vi "VFD.vi"() -> (0 "GS1 Communication Error Out":errorcluster)   [LabVIEW 2017]
uses:
  XDataNode.xnode
panel:
  in  "GS1 Communication Error In":errorcluster
  out "Iteration Duration":i64
  out "Finished Late? [i-1]":bool
  out "TCHX Initializaton Error":errorcluster
  out "TCHX Initialization Loop Time (ms)":u32
  out "CTAH Initializaton Error":errorcluster
  out "CTAH Initialization Loop Time (ms)":u32
  out "Pump Initializaton Error":errorcluster
  out "Pump Initialization Loop Time (ms)":u32
  in  "Starting Address":u16
  out "Holding Registers":u16[](array[numeric])
  out "error out":errorcluster
  out "VISA resource name out":refnum<visa-resource-name>
  out "400001":u16
  out "error out":errorcluster
  # "Troubleshooting Modbus communication using third-party VIs and native I/O Server"
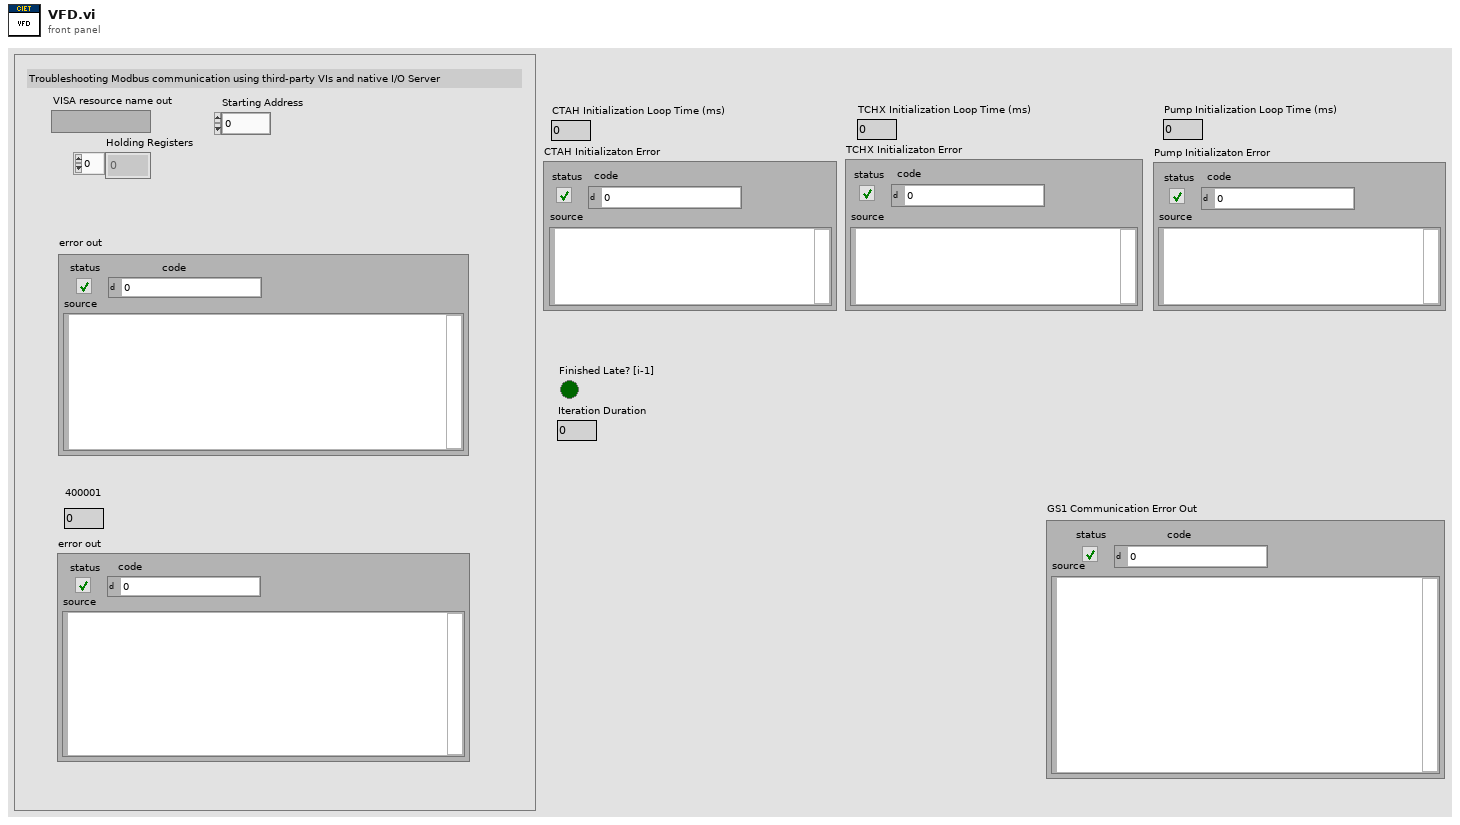
[diagram p1: front panel]
types:
  T1 = cluster{"Mode":enum16{"RTU", "ASCII"}, "Slave Address":u8}
  T2 = cluster{"Expected End [f-1]":u64, "Actual End [f-1]":u64, "Finished Late? [f-1]":bool, "Expected End [i-1]":u64, "Actual End [i-1]":u64, "Finished Late? [i-1]":bool, "Expected Start [i]":u64, "Actual Start [i]":u64, "Expected Start [f]":u64, "Actual Start [f]":u64, "Source Name":string, "Structure Name":string, "Period":i64, "Deadline":i64, "Offset":i64, "Start":i64, "Priority":i32, "Timeout":i32, "Mode":enum32{"No Change", "Process missed periods, maintain original phase", "Discard missed periods, maintain original phase", "Process missed periods, ignore original phase", "Discard missed periods, ignore original phase"}, "Wakeup Reason":enum32{"Normal", "Aborted", "Asynchronous wakeup", "Timing source error", "Timed loop error", "Timeout"}, "Error":errorcluster, "Source Type":string, "Secondary Source Type":string, "Global End Time":u64, "Global Start Time":u64, "Frame Duration":u64, "Iteration Duration":u64, "Assigned CPU":i32, "I/O Scan Engine Mode":u32}
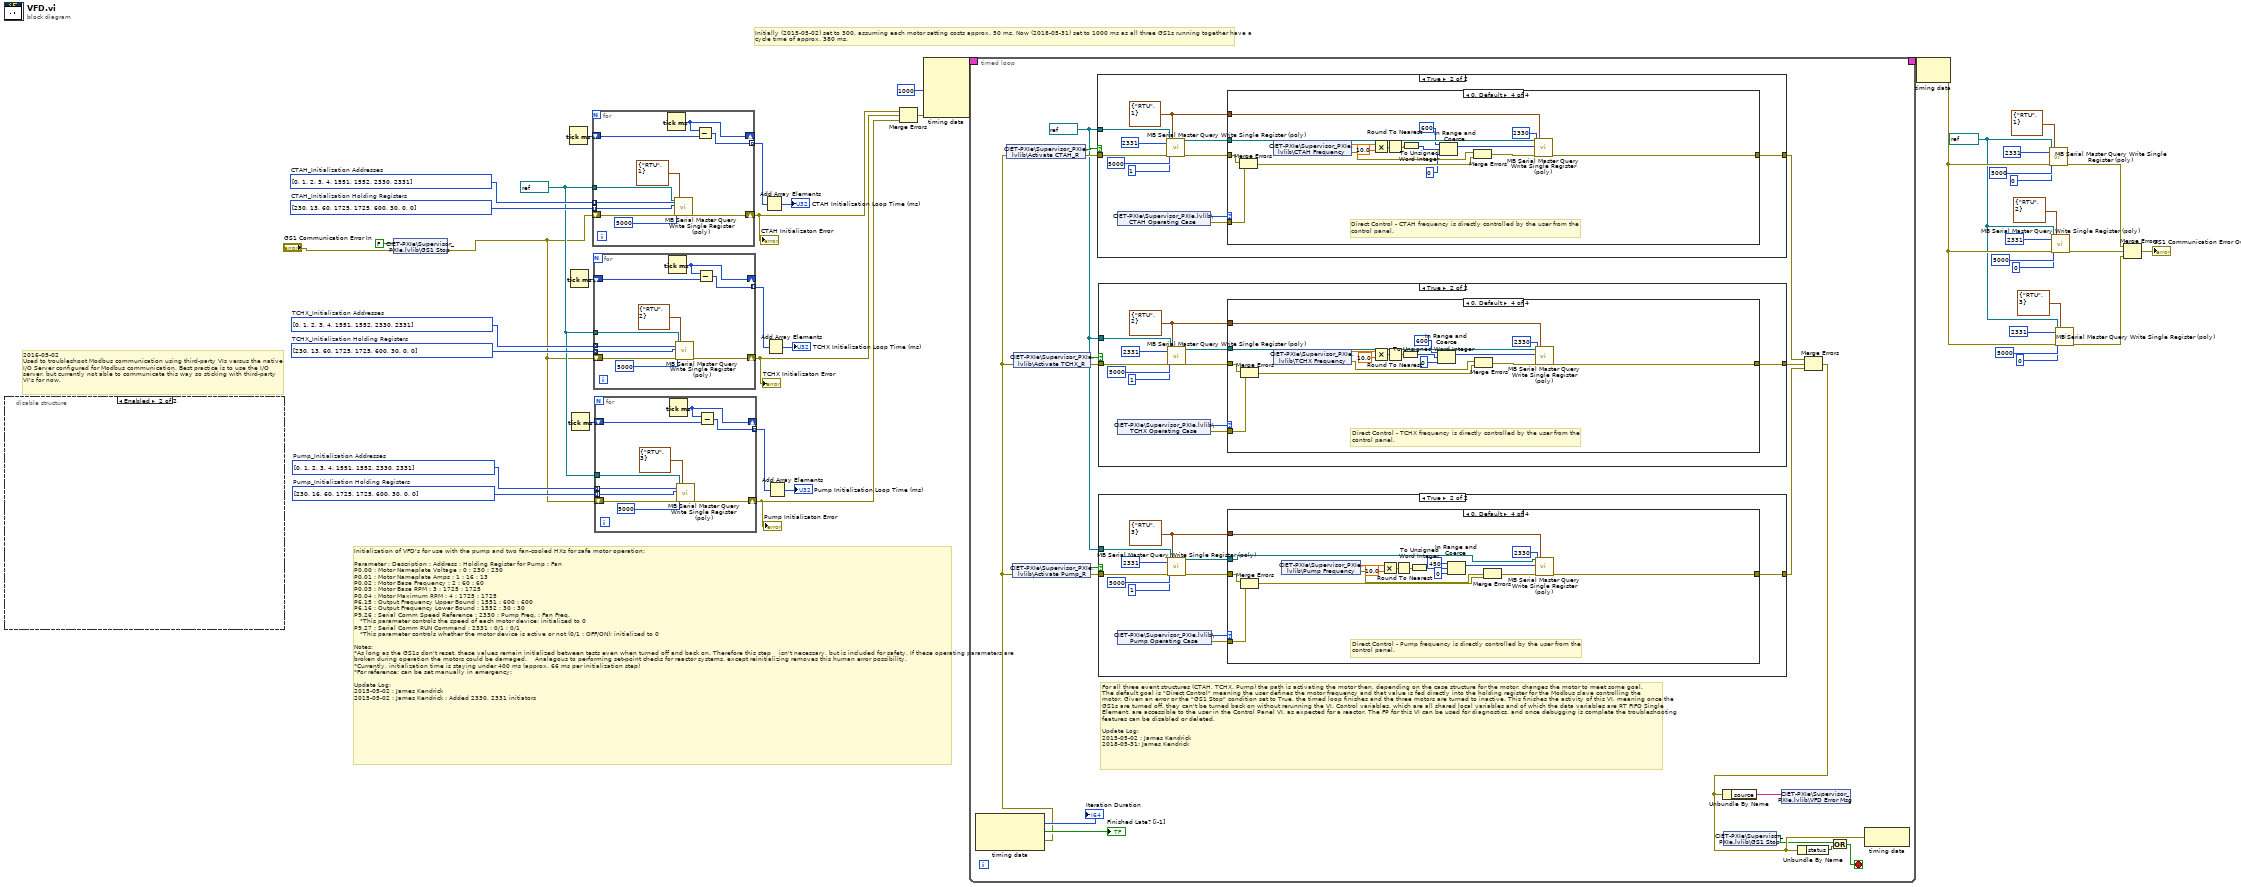
[diagram p0: block diagram]
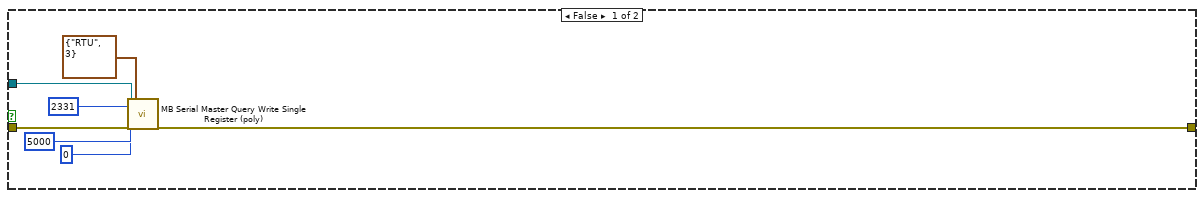
[diagram p2: hidden frame]
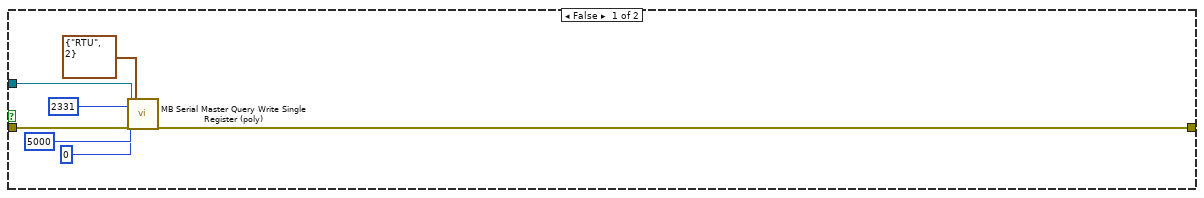
[diagram p6: hidden frame]
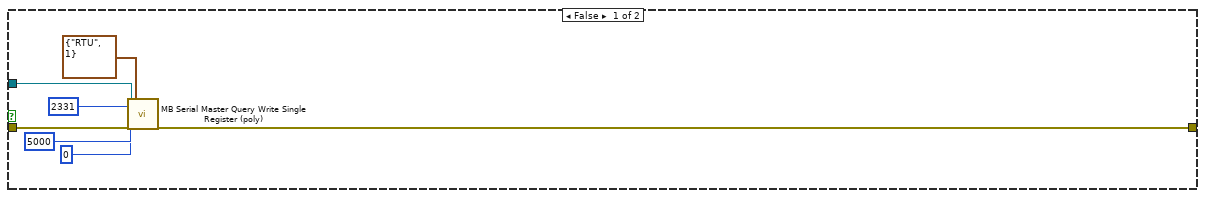
[diagram p10: hidden frame]
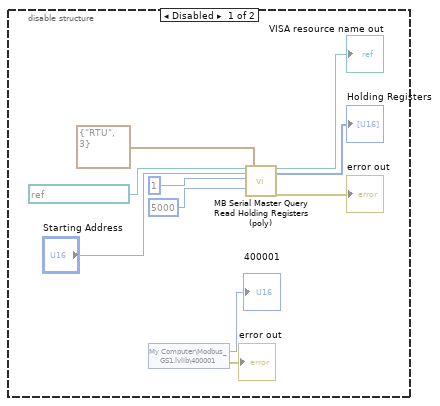
[diagram p14: hidden frame]
diagram:
  w7 = refnum<visa-resource-name> "VFD" ("VISA resource name")
  w8 = refnum<visa-resource-name> "VFD" ("VISA resource name")
  w30 = u16[] [230, 13, 60, 1725, 1725, 600, 30, 0, 0]  # TCHX_Initialization Holding Registers
  w31 = u16[] [0, 1, 2, 3, 4, 1551, 1552, 2330, 2331]  # TCHX_Initialization Addresses
  w35 = u16[] [230, 13, 60, 1725, 1725, 600, 30, 0, 0]  # CTAH_Initialization Holding Registers
  w36 = u16[] [0, 1, 2, 3, 4, 1551, 1552, 2330, 2331]  # CTAH_Initialization Addresses
  w43 = u16[] [230, 16, 60, 1725, 1725, 600, 30, 0, 0]  # Pump_Initialization Holding Registers
  w44 = u16[] [0, 1, 2, 3, 4, 1551, 1552, 2330, 2331]  # Pump_Initialization Addresses
  # "Initially (2015-05-02) set to 300, assuming each motor setting costs approx. 50 ms. Now (2018-05-31) set to 1000 ms as all three GS1s running together have a \ncycle time of approx. 380 ms."
  # "2016-05-02\nUsed to troubleshoot Modbus communication using third-party VIs versus the native\nI/O Server configured for Modbus communication. Best practice is to use the I/O \nserver, but currently not able to communicate this way so sticking with third-party \nVI's for now."
  # "Initialization of VFD's for use with the pump and two fan-cooled HXs for safe motor operation:\n\nParameter : Description : Address : Holding Register for Pump : Fan\nP0.00 : Motor Nameplate Voltage : 0 : 230 : 230\nP0.01 : Motor Nameplate Amps : 1 : 16 : 13\nP0.02 : Motor Base Frequency : 2 : 60 : 60\nP0.03 : Motor Base RPM : 3 : 1725 : 1725\nP0.04 : Motor Maximum RPM : 4 : 1725 : 1725\nP6.15 : Output Frequency Upper Bound : 1551 : 600 : 600\nP6.16 : Output Frequency Lower Bound : 1552 : 30 : 30\nP9.26 : Serial Comm Speed Reference : 2330 : Pump Freq. : Fan Freq. \n   *This parameter controls the speed of each motor device; initialized to 0\nP9.27 : Serial Comm RUN Command : 2331 : 0/1 : 0/1\n   *This parameter controls whether the motor device is active or not (0/1 : OFF/ON); initialized to 0\n\nNotes:\n*As long as the GS1s don't reset, these values remain initialized between tests even when turned off and back on. Therefore this step    isn't necessary, but is included for safety. If these operating parameters are broken during operation the motors could be damaged.    Analagous to performing set-point checks for reactor systems, except reinitializing removes this human error possibility.\n*Currently, initialization time is staying under 400 ms (approx. 66 ms per initialization step)\n*For reference; can be set manually in emergency:\n\nUpdate Log:\n2015-05-02 : James Kendrick \n2015-05-02 : James Kendrick : Added 2330, 2331 initiators"
  n1 = disable-structure shown="Enabled" {
    frame Disabled {
      n2 = shared-variable "My Computer\\Modbus_GS1.lvlib\\400001"() -> (→"400001":u16, error out=→"error out":errorcluster)  [unwired: 1 in]
      n3 = call "MB Serial Master Query Read Holding Registers (poly).vi"("VISA resource name"=refnum<visa-resource-name> "GS1_AC_Drive", "Starting Address"="Starting Address", "Quantity"=u16 1, "Timeout"=u32 5000, "Serial Parameters"=T1 {"Mode"=enum."RTU", "Slave Address"=3}) -> ("VISA resource name out"=→"VISA resource name out":refnum<visa-resource-name>, "Holding Registers"=→"Holding Registers":u16[], "error out"=→"error out":errorcluster)  [unwired: 11 in, 1 out]
    }
    frame Enabled {
    }
  }
  n4 = shared-variable "CIET-PXIe\\Supervisor_PXIe.lvlib\\GS1 Stop"(FALSE ("GS1 Stop"), error in="GS1 Communication Error In") -> (error out=w2:errorcluster)
  n5 = Tick Count (ms)() -> (millisecond timer value=w34:u32)
  n6 = Tick Count (ms)() -> (millisecond timer value=w29:u32)
  n7 = Tick Count (ms)() -> (millisecond timer value=w42:u32)
  n8 = for {
    shift-right: [w62] -> w16
    shift-left: w2 -> [w63]
    tunnel: w36 -> [w61] mode=indexing
    tunnel: w35 -> [w60] mode=indexing
    shift-right: [w57] -> _
    shift-left: w34 -> [w59]
    tunnel: [w58] -> w33 mode=indexing
    tunnel: w8 -> [w56]
    n9 = Tick Count (ms)() -> (millisecond timer value=w57:u32)
    n10 = call "MB Serial Master Query Write Single Register (poly).vi"("VISA resource name"=w56, "Address"=w61, "Holding Register"=w60, "Timeout"=u32 5000, "error in"=w63, "Serial Parameters"=T1 {"Mode"=enum."RTU", "Slave Address"=1}) -> ("error out"=w62:errorcluster)  [unwired: 11 in, 2 out]
    n11 = Subtract(x=w57, y=w59) -> (x-y=w58:u32)
  }
  "CTAH Initializaton Error" <- w16
  n12 = for {
    shift-right: [w72] -> w10
    shift-left: w2 -> [w73]
    tunnel: w31 -> [w71] mode=indexing
    tunnel: w30 -> [w70] mode=indexing
    shift-right: [w67] -> _
    shift-left: w29 -> [w69]
    tunnel: [w68] -> w28 mode=indexing
    tunnel: w8 -> [w66]
    n13 = Tick Count (ms)() -> (millisecond timer value=w67:u32)
    n14 = call "MB Serial Master Query Write Single Register (poly).vi"("VISA resource name"=w66, "Address"=w71, "Holding Register"=w70, "Timeout"=u32 5000, "error in"=w73, "Serial Parameters"=T1 {"Mode"=enum."RTU", "Slave Address"=2}) -> ("error out"=w72:errorcluster)  [unwired: 11 in, 2 out]
    n15 = Subtract(x=w67, y=w69) -> (x-y=w68:u32)
  }
  "TCHX Initializaton Error" <- w10
  n16 = for {
    shift-right: [w82] -> w9
    shift-left: w2 -> [w83]
    tunnel: w44 -> [w81] mode=indexing
    tunnel: w43 -> [w80] mode=indexing
    shift-right: [w77] -> _
    shift-left: w42 -> [w79]
    tunnel: [w78] -> w41 mode=indexing
    tunnel: w8 -> [w76]
    n17 = Tick Count (ms)() -> (millisecond timer value=w77:u32)
    n18 = call "MB Serial Master Query Write Single Register (poly).vi"("VISA resource name"=w76, "Address"=w81, "Holding Register"=w80, "Timeout"=u32 5000, "error in"=w83, "Serial Parameters"=T1 {"Mode"=enum."RTU", "Slave Address"=3}) -> ("error out"=w82:errorcluster)  [unwired: 11 in, 2 out]
    n19 = Subtract(x=w77, y=w79) -> (x-y=w78:u32)
  }
  "Pump Initializaton Error" <- w9
  n20 = Add Array Elements(numeric array=w33) -> (sum=→"CTAH Initialization Loop Time (ms)":u32)
  n21 = Add Array Elements(numeric array=w28) -> (sum=→"TCHX Initialization Loop Time (ms)":u32)
  n22 = Add Array Elements(numeric array=w41) -> (sum=→"Pump Initialization Loop Time (ms)":u32)
  n23 = Merge Errors(w16, w10, w9) -> (w17:errorcluster)
  n24 = node-c288(i64 1000 ("Pump Control Period (ms)"), w17) -> (w39:T2)  [unwired: 3 in]
  n25 = timed-loop {
    timing: w39 -> [_]
    timing-out: [_] -> w38
    stop <- w98 stop-if-true
    w88 = refnum<visa-resource-name> "VFD" ("VISA resource name")
    # "For all three event structures (CTAH, TCHX, Pump) the path is activating the motor then, depending on the case structure for the motor, changes the motor to meet some goal. \nThe default goal is \"Direct Control\" meaning the user defines the motor frequency and that value is fed directly into the holding register for the Modbus slave controlling the \nmotor. Given an error or the \"GS1 Stop\" condition set to True, the timed loop finishes and the three motors are turned to inactive. This finishes the activity of this VI, meaning once the\nGS1s are turned off, they can't be turned back on without rerunning the VI. Control variables, which are all shared local variables and of which the data variables are RT FIFO Single\nElement, are accessible to the user in the Control Panel VI, as expected for a reactor. The FP for this VI can be used for diagnostics, and once debugging is complete the troubleshooting\nfeatures can be disabled or deleted.  \n\nUpdate Log:\n2015-05-02 : James Kendrick\n2018-05-31: James Kendrick"
    n26 = node-c288() -> (→"Iteration Duration":i64, →"Finished Late? [i-1]":bool, w92:errorcluster)  [unwired: 1 in]
    n27 = shared-variable "CIET-PXIe\\Supervisor_PXIe.lvlib\\Activate CTAH_R"(error in=w92) -> (w102:bool, error out=w101:errorcluster)
    n28 = shared-variable "CIET-PXIe\\Supervisor_PXIe.lvlib\\Activate Pump_R"(error in=w92) -> (w95:bool, error out=w94:errorcluster)
    n29 = shared-variable "CIET-PXIe\\Supervisor_PXIe.lvlib\\Activate TCHX_R"(error in=w92) -> (w97:bool, error out=w96:errorcluster)
    n30 = case shown="True" w102 {
      tunnel: w101 -> [w176 w186]
      tunnel: [w175 w182] -> w91
      tunnel: w88 -> [w174 w181]
      frame False {
        n31 = call "MB Serial Master Query Write Single Register (poly).vi"("VISA resource name"=w174, "Address"=u16 2331, "Holding Register"=u16 0, "Timeout"=u32 5000, "error in"=w176, "Serial Parameters"=T1 {"Mode"=enum."RTU", "Slave Address"=1}) -> ("error out"=w175:errorcluster)  [unwired: 11 in, 2 out]
      }
      frame True {
        w180 = T1 {"Mode"=enum."RTU", "Slave Address"=1} ("Serial Parameters")
        n32 = shared-variable "CIET-PXIe\\Supervisor_PXIe.lvlib\\CTAH Operating Case"() -> (w184:i32, error out=w183:errorcluster)  [unwired: 1 in]
        n33 = call "MB Serial Master Query Write Single Register (poly).vi"("VISA resource name"=w181, "Address"=u16 2331, "Holding Register"=u16 1, "Timeout"=u32 5000, "error in"=w186, "Serial Parameters"=w180) -> ("VISA resource name out"=w185:refnum<visa-resource-name>, "error out"=w187:errorcluster)  [unwired: 11 in, 1 out]
        n34 = case shown="0, Default" w184 {
          tunnel: w187 -> [_ _ _ w206]
          tunnel: w185 -> [_ _ _ w207]
          tunnel: w183 -> [_ _ _ w205]
          tunnel: [_ _ _ w201] -> w182
          tunnel: w180 -> [_ _ _ w200]
          frame 1 {
            # "CTAH Outlet Temp: Feedback - CTAH frequency is determined by a\ncontrol function to hold the outlet temperature of the CTAH \nconstant."
          }
          frame 2 {
            # "Load Following - CTAH frequency is controlled to make the CTAH heat removal power\nto equal a user specified value through satisfying the equation: m_dot*c_P*(T_in - T_out)"
          }
          frame 3 {
            # "Dynamic Forcing - CTAH frequency is defined by a waveform function to drive the \nCTAH frequency and thus mass flow rate in a dynamic pattern, such as a square wave,\nsine wave, or other function as defined by the user.\n\nUser inputs to include:\nCTAH frequency set point (used as signal offset)\nSignal amplitude\nSignal frequency\nSignal type: sine, square, others?"
          }
          frame 0, Default {
            # "Direct Control - CTAH frequency is directly controlled by the user from the\ncontrol panel."
            n35 = Merge Errors(w206, w205) -> (w202:errorcluster)
            n36 = shared-variable "CIET-PXIe\\Supervisor_PXIe.lvlib\\CTAH Frequency"() -> (w197:sgl, error out=w198:errorcluster)  [unwired: 1 in]
            n37 = Multiply(x=w197, y=sgl 10.0) -> (x*y=w199:sgl)
            n38 = Round To Nearest(number=w199) -> (nearest integer value=w196:sgl)
            n39 = To Unsigned Word Integer(number=w196) -> (unsigned 16bit integer=w194:u16)
            n40 = In Range and Coerce(upper limit=u16 600, x=w194, lower limit=u16 0) -> (coerced(x)=w193:u16)  [unwired: 1 out]
            n41 = Merge Errors(w198, w202) -> (w203:errorcluster)
            n42 = call "MB Serial Master Query Write Single Register (poly).vi"("VISA resource name"=w207, "Address"=u16 2330, "Holding Register"=w193, "error in"=w203, "Serial Parameters"=w200) -> ("error out"=w201:errorcluster)  [unwired: 12 in, 2 out]
          }
        }
      }
    }
    n43 = case shown="True" w97 {
      tunnel: w96 -> [w141 w151]
      tunnel: [w140 w147] -> w90
      tunnel: w88 -> [w139 w146]
      frame False {
        n44 = call "MB Serial Master Query Write Single Register (poly).vi"("VISA resource name"=w139, "Address"=u16 2331, "Holding Register"=u16 0, "Timeout"=u32 5000, "error in"=w141, "Serial Parameters"=T1 {"Mode"=enum."RTU", "Slave Address"=2}) -> ("error out"=w140:errorcluster)  [unwired: 11 in, 2 out]
      }
      frame True {
        w145 = T1 {"Mode"=enum."RTU", "Slave Address"=2} ("Serial Parameters")
        n45 = shared-variable "CIET-PXIe\\Supervisor_PXIe.lvlib\\TCHX Operating Case"() -> (w149:i32, error out=w148:errorcluster)  [unwired: 1 in]
        n46 = call "MB Serial Master Query Write Single Register (poly).vi"("VISA resource name"=w146, "Address"=u16 2331, "Holding Register"=u16 1, "Timeout"=u32 5000, "error in"=w151, "Serial Parameters"=w145) -> ("VISA resource name out"=w150:refnum<visa-resource-name>, "error out"=w152:errorcluster)  [unwired: 11 in, 1 out]
        n47 = case shown="0, Default" w149 {
          tunnel: w152 -> [_ _ _ w171]
          tunnel: w150 -> [_ _ _ w172]
          tunnel: w148 -> [_ _ _ w170]
          tunnel: [_ _ _ w166] -> w147
          tunnel: w145 -> [_ _ _ w165]
          frame 1 {
            # "TCHX Outlet Temp: Feedback - TCHX frequency is determined by a\ncontrol function to hold the outlet temperature of the TCHX \nconstant."
          }
          frame 2 {
            # "Freezing Event - TCHX frequency is adjust to simulate a freezing transient or freeze\nevent within the TCHX, compromising the heat transfer path from the core to\nenvironment during a transient without use of the pump/CTAH."
          }
          frame 3 {
            # "Dynamic Forcing - TCHX frequency is defined by a waveform function to drive the \nTCHX frequency and thus mass flow rate in a dynamic pattern, such as a square wave,\nsine wave, or other function as defined by the user.\n\nUser inputs to include:\nTCHX frequency set point (used as signal offset)\nSignal amplitude\nSignal frequency\nSignal type: sine, square, others?"
          }
          frame 0, Default {
            # "Direct Control - TCHX frequency is directly controlled by the user from the\ncontrol panel."
            n48 = Merge Errors(w171, w170) -> (w167:errorcluster)
            n49 = shared-variable "CIET-PXIe\\Supervisor_PXIe.lvlib\\TCHX Frequency"() -> (w164:sgl, error out=w160:errorcluster)  [unwired: 1 in]
            n50 = Multiply(x=w164, y=sgl 10.0) -> (x*y=w163:sgl)
            n51 = Round To Nearest(number=w163) -> (nearest integer value=w162:sgl)
            n52 = To Unsigned Word Integer(number=w162) -> (unsigned 16bit integer=w158:u16)
            n53 = In Range and Coerce(upper limit=u16 600, x=w158, lower limit=u16 0) -> (coerced(x)=w159:u16)  [unwired: 1 out]
            n54 = Merge Errors(w160, w167) -> (w168:errorcluster)
            n55 = call "MB Serial Master Query Write Single Register (poly).vi"("VISA resource name"=w172, "Address"=u16 2330, "Holding Register"=w159, "error in"=w168, "Serial Parameters"=w165) -> ("error out"=w166:errorcluster)  [unwired: 12 in, 2 out]
          }
        }
      }
    }
    n56 = case shown="True" w95 {
      tunnel: w94 -> [w106 w116]
      tunnel: [w105 w112] -> w89
      tunnel: w88 -> [w104 w111]
      frame False {
        n57 = call "MB Serial Master Query Write Single Register (poly).vi"("VISA resource name"=w104, "Address"=u16 2331, "Holding Register"=u16 0, "Timeout"=u32 5000, "error in"=w106, "Serial Parameters"=T1 {"Mode"=enum."RTU", "Slave Address"=3}) -> ("error out"=w105:errorcluster)  [unwired: 11 in, 2 out]
      }
      frame True {
        w110 = T1 {"Mode"=enum."RTU", "Slave Address"=3} ("Serial Parameters")
        n58 = shared-variable "CIET-PXIe\\Supervisor_PXIe.lvlib\\Pump Operating Case"() -> (w114:i32, error out=w113:errorcluster)  [unwired: 1 in]
        n59 = call "MB Serial Master Query Write Single Register (poly).vi"("VISA resource name"=w111, "Address"=u16 2331, "Holding Register"=u16 1, "Timeout"=u32 5000, "error in"=w116, "Serial Parameters"=w110) -> ("VISA resource name out"=w115:refnum<visa-resource-name>, "error out"=w117:errorcluster)  [unwired: 11 in, 1 out]
        n60 = case shown="0, Default" w114 {
          tunnel: w117 -> [_ _ _ w137]
          tunnel: w115 -> [_ _ _ w127]
          tunnel: w113 -> [_ _ _ w136]
          tunnel: [_ _ _ w132] -> w112
          tunnel: w110 -> [_ _ _ w126]
          frame 1 {
            # "Mass Flow Rate: Feedback - Pump frequency is controlled through \na closed feedback to match a specified mass flow rate defined by \nthe user on the control panel."
          }
          frame 2 {
            # "Mass Flow Rate: Ramp - Pump frequency is controlled through a control function that\ncontrols the rate of change of the mass flow rate that the user specifies on the control\npanel to match a user desired final mass flow rate."
          }
          frame 3 {
            # "Dynamic Forcing - Pump frequency is defined by a waveform function to drive the \npump frequency and thus mass flow rate in a dynamic pattern, such as a square wave,\nsine wave, or other function as defined by the user.\n\nUser inputs to include:\nPump frequency set point (used as signal offset)\nSignal amplitude\nSignal frequency\nSignal type: sine, square, others?"
          }
          frame 0, Default {
            # "Direct Control - Pump frequency is directly controlled by the user from the\ncontrol panel."
            n61 = Merge Errors(w137, w136) -> (w133:errorcluster)
            n62 = shared-variable "CIET-PXIe\\Supervisor_PXIe.lvlib\\Pump Frequency"() -> (w124:sgl, error out=w128:errorcluster)  [unwired: 1 in]
            n63 = Multiply(x=w124, y=sgl 10.0) -> (x*y=w125:sgl)
            n64 = Round To Nearest(number=w125) -> (nearest integer value=w122:sgl)
            n65 = To Unsigned Word Integer(number=w122) -> (unsigned 16bit integer=w121:u16)
            n66 = In Range and Coerce(upper limit=u16 450, x=w121, lower limit=u16 0) -> (coerced(x)=w129:u16)  [unwired: 1 out]
            n67 = Merge Errors(w128, w133) -> (w134:errorcluster)
            n68 = call "MB Serial Master Query Write Single Register (poly).vi"("VISA resource name"=w127, "Address"=u16 2330, "Holding Register"=w129, "error in"=w134, "Serial Parameters"=w126) -> ("error out"=w132:errorcluster)  [unwired: 12 in, 2 out]
          }
        }
      }
    }
    n69 = shared-variable "CIET-PXIe\\Supervisor_PXIe.lvlib\\GS1 Stop"() -> (w85:bool)  [unwired: 1 in, 1 out]
    n70 = Merge Errors(w91, w90, w89) -> (w87:errorcluster)
    n71 = Unbundle By Name(w87) -> ("source"=w86:string)
    n72 = shared-variable "CIET-PXIe\\Supervisor_PXIe.lvlib\\VFD Error Msg"(w86) -> ()  [unwired: 1 in, 1 out]
    n73 = Unbundle By Name(w87) -> ("status"=w93:bool)
    n74 = Or(x=w85, y=w93) -> (x .or. y?=w98:bool)
    n75 = node-c288(w87) -> ()  [unwired: 1 out]
  }
  n76 = node-c288(w38) -> (w11:errorcluster)
  n77 = call "MB Serial Master Query Write Single Register (poly).vi"("VISA resource name"=w7, "Address"=u16 2331, "Holding Register"=u16 0, "Timeout"=u32 5000, "error in"=w11, "Serial Parameters"=T1 {"Mode"=enum."RTU", "Slave Address"=1}) -> ("error out"=w13:errorcluster)  [unwired: 11 in, 2 out]
  n78 = call "MB Serial Master Query Write Single Register (poly).vi"("VISA resource name"=w7, "Address"=u16 2331, "Holding Register"=u16 0, "Timeout"=u32 5000, "error in"=w11, "Serial Parameters"=T1 {"Mode"=enum."RTU", "Slave Address"=2}) -> ("error out"=w14:errorcluster)  [unwired: 11 in, 2 out]
  n79 = call "MB Serial Master Query Write Single Register (poly).vi"("VISA resource name"=w7, "Address"=u16 2331, "Holding Register"=u16 0, "Timeout"=u32 5000, "error in"=w11, "Serial Parameters"=T1 {"Mode"=enum."RTU", "Slave Address"=3}) -> ("error out"=w12:errorcluster)  [unwired: 11 in, 2 out]
  n80 = Merge Errors(w13, w14, w12) -> (→"GS1 Communication Error Out":errorcluster)
